vi "Updater Back Up Database.vi"(6 "DEBUG? (f)":bool, 8 "error in (no error)":errorcluster, 11 "Database Path (empty)":path) -> (0 "error out":errorcluster, 3 "dup Database Path":path)   [LabVIEW 2011]
uses:
  Summitek EXT/OpenG EXT/file/file.llb/Strip Path Extension - String__ogtk.vi
  Summitek EXT/OpenG EXT/file/file.llb/Convert File Extension (String)__ogtk.vi
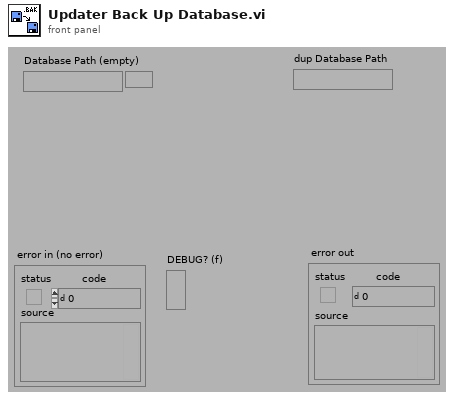
[diagram p1: front panel]
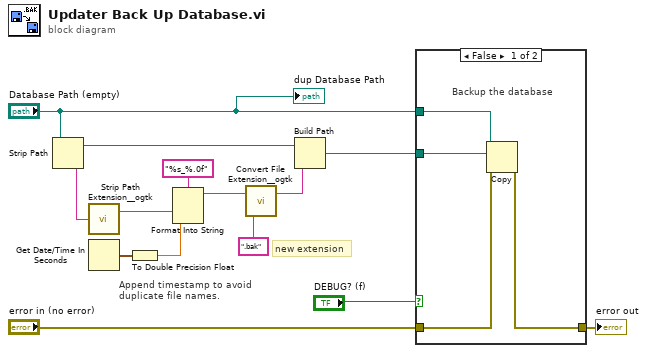
[diagram p0: block diagram]
diagram:
  # "new extension"
  # "Append timestamp to avoid \nduplicate file names."
  n1 = Strip Path(path="Database Path (empty)") -> (stripped path=w12:path, name=w8:string)
  n2 = call-poly "Strip Path Extension__ogtk.vi"("path"=w8) -> ("root"=w7:string)  [unwired: 1 out]
  n3 = Get Date/Time In Seconds() -> (seconds since 1Jan1904=w9:timestamp)
  n4 = To Double Precision Float(number=w9) -> (double precision float=w6:dbl)
  n5 = Format Into String(format string="%s_%.0f" ("name or relative path"), w7, w6) -> (resulting string=w5:string)  [unwired: 2 in, 1 out]
  n6 = call-poly "Convert File Extension__ogtk.vi"("new ending (none)"=".bak" ("name or relative path"), "file name"=w5) -> ("new filename"=w3:string)  [unwired: 1 out]
  n7 = Build Path(base path=w12, name or relative path=w3) -> (appended path=w14:path)
  n8 = case shown="False" "DEBUG? (f)" {
    tunnel: w14 -> [w18 _]
    tunnel: "Database Path (empty)" -> [w17 _]
    tunnel: "error in (no error)" -> [w16 w19]
    tunnel: [w15 w19] -> w10
    frame False {
      # "Backup the database"
      n9 = Copy(8:w16, 10:w18, 11:w17) -> (0:w15:errorcluster)  [unwired: 4 out]
    }
    frame True {
    }
  }
  "error out" <- w10
  "dup Database Path" <- "Database Path (empty)"
